vi "GlobalVars.vi"() -> ()   [LabVIEW 2016]
panel:
  out "Escaped":bool
  out "Connected":bool
  out "Disconnect":bool
  out "Msg Seq No":u8
  out "Msg Send Q Name":string
  out "Msg Send Q Ref":T1
  out "Hdr Size":u8
  out "Max Msg Len":u16
  out "Exit":bool
  out "Msg Recv Q Name":string
  out "Msg Recv Q Ref":T1
  out "Msg Len":u32
  out "Msg State":string
  out "Msg Idx":u32
  out "Message":u8[](array[numeric])
  # "Constants for header size and maximum message length are\n set in BristolExample.vi, sequence 0 (Initialize)."
  # "Queue to hold messages received on the serial port."
  # "Queue to hold messages to be sent out the serial port."
  # "Sequence number to be sent with next message sent.  Is incremented by one on each send."
  # "Current state of message parser."
  # "Indicates that the previous character recieved was the escape character."
  # "Parser builds output into Message, inserts data at Msg Idx position\nand keeps track of the message length in Msg Len."
  # "Exit flag is set when user selectes exit - it is used to control the termination of tasks.\nConnected indicates the serial port is open.  Disconnect is set when the user requests\nthe close of the serial port - the serial manager tasks will terminate if this flag is set."
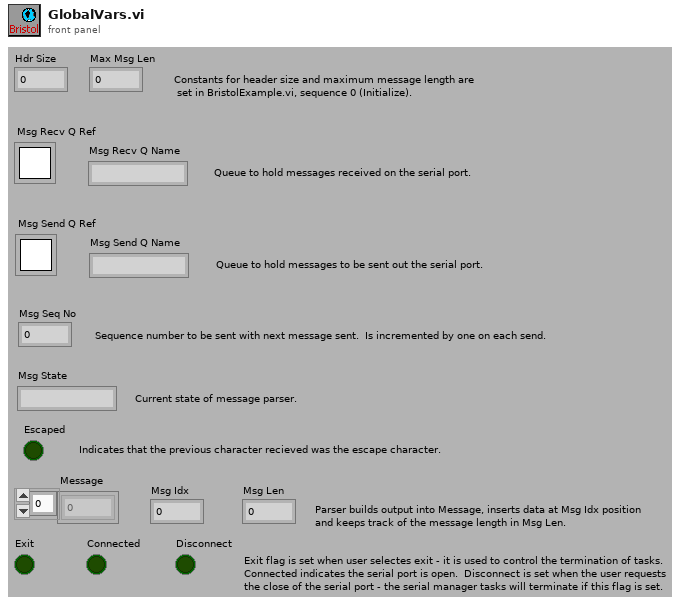
[diagram p1: front panel]
types:
  T1 = typedef "Queue RefNum" = refnum<k1>
diagram:
